vi "RT Loop - Image Acquisition and Processing.vi"(8 "error in (no error)":errorcluster, 9 "FPGA VI Reference":T1, 10 "Vision Cmd Queue":refnum<queue>, 11 "Message Handling Queue":refnum<queue>) -> ()   [LabVIEW 2018]
doc: "Executes the sequence sent from the main UI."
uses:
  controls/Sequence Engine State.ctl
  controls/FPGA VI Reference.ctl
  <vilib>/rvi/interface/nirviReadWriteControl/nirviReadWriteControl.xnode
  NiFpgaLv.dll
  <vilib>/Utility/error.llb/Error Cluster From Error Code.vi
  <vilib>/rvi/interface/Simulation/niFpgaSimulationCallBeginRW.vi
  <vilib>/rvi/errors/niLvFpgaAdjustHostInterfaceError.vi
  support/Message Queue/Message Cluster.ctl
  support/Message Queue/Message Queue.lvlib
  Globals/Global - All RT Loop Stop.vi
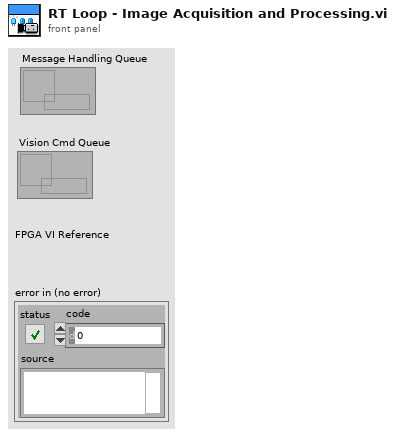
[diagram p1: front panel]
types:
  T1 = typedef "FPGA VI Reference.ctl" = refnum<k20>
  T2 = typedef "Message Queue.lvlib/Message Cluster.ctl" = cluster{"Message":string, "Message Data":variant}
  T3 = typedef "Sequence Engine State.ctl" = enum16{"Idle", "Running", "Stop", "Pause", "Resume", "Load Sequence"}
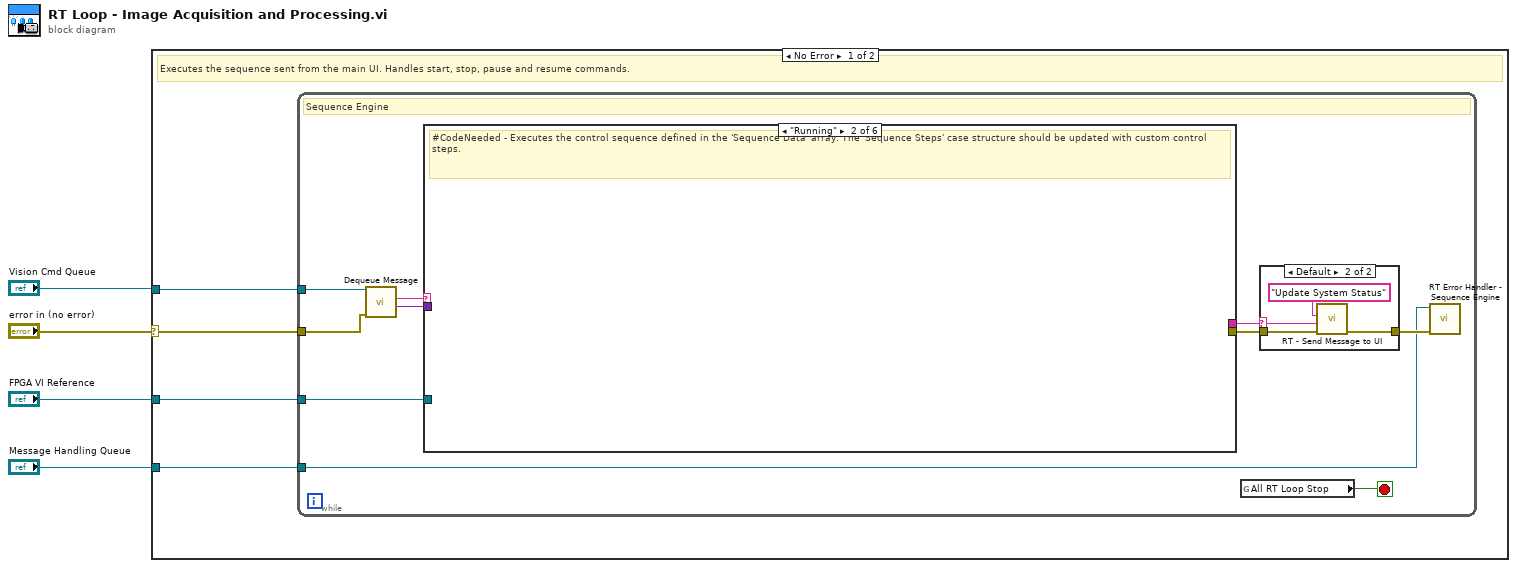
[diagram p0: block diagram]
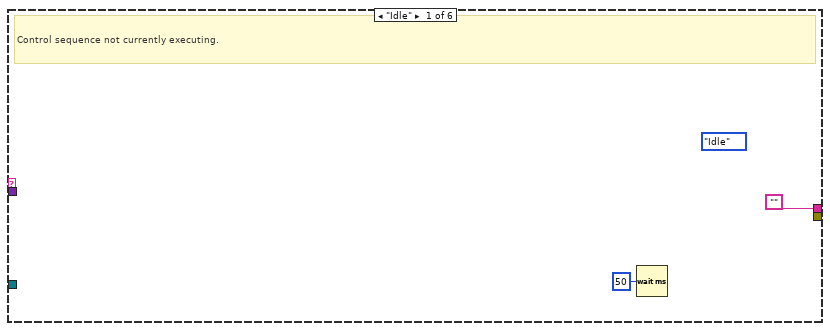
[diagram p3: hidden frame]
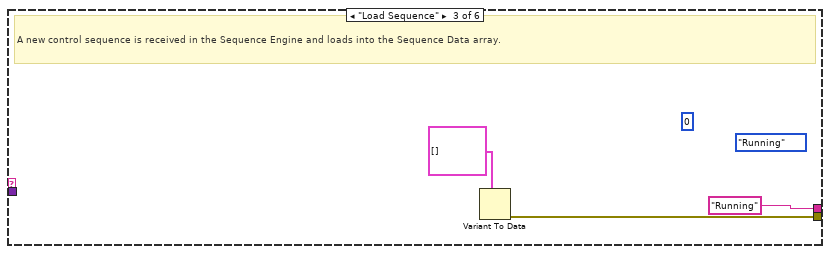
[diagram p4: hidden frame]
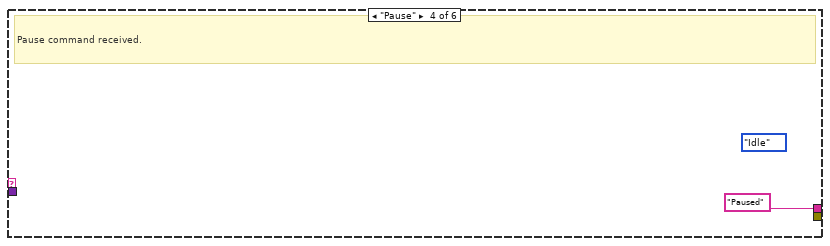
[diagram p5: hidden frame]
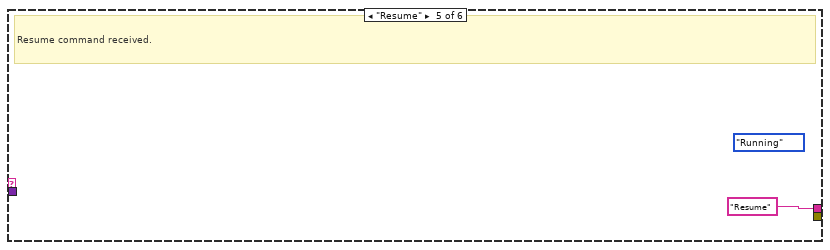
[diagram p6: hidden frame]
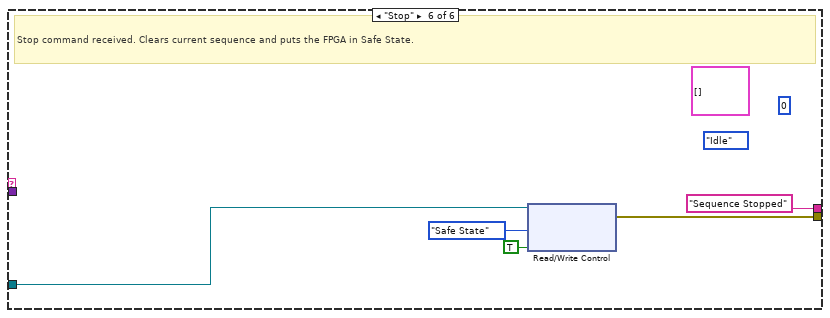
[diagram p7: hidden frame]
diagram:
  n1 = case shown="No Error" "error in (no error)" {
    selector: "error in (no error)" -> [w5 _]
    tunnel: "Message Handling Queue" -> [w8 _]
    tunnel: "Vision Cmd Queue" -> [w7 _]
    tunnel: "FPGA VI Reference" -> [w6 _]
    frame No Error {
      # "Executes the sequence sent from the main UI. Handles start, stop, pause and resume commands."
      n2 = while "Sequence Engine" {
        tunnel: w7 -> [w12]
        tunnel: w6 -> [w18]
        tunnel: w8 -> [w15]
        tunnel: w5 -> [w11]
        stop <- w14 stop-if-true
        # "Sequence Engine"
        n3 = call "Dequeue Message.vi"("error in (no error)"=w11, "Message Queue"=w12) -> ("Message Data"=w9:variant, "Message"=w10:string)  [unwired: 6 in, 2 out]
        n4 = case shown="\"Running\"" w10 {
          tunnel: w18 -> [_ _ _ _ _ w43]
          tunnel: [_ _ w29 _ _ w42] -> w17
          tunnel: ["" ("f") _ "Running" ("f") "Paused" "Resume" ("f") "Sequence Stopped"] -> w13
          tunnel: w9 -> [_ _ _ _ _ _]
          frame "Idle" {
            w25 = Sequence_Engine_State."Idle" ("Sequence Engine State")
            # "Control sequence not currently executing."
            n5 = Wait (ms)(milliseconds to wait=u32 50) -> ()  [unwired: 1 out]
          }
          frame "Running" {
            # "#CodeNeeded - Executes the control sequence defined in the 'Sequence Data' array. The 'Sequence Steps' case structure should be updated with custom control steps."
          }
          frame "Load Sequence" {
            w31 = 0 ("Current Step")
            w30 = Sequence_Engine_State."Running" ("Sequence Engine State")
            # "A new control sequence is received in the Sequence Engine and loads into the Sequence Data array."
            n6 = Variant To Data(type=T2[] []) -> (data=w32:T2[], error out=w29:errorcluster)  [unwired: 2 in]
          }
          frame "Pause" {
            w34 = Sequence_Engine_State."Idle" ("Sequence Engine State")
            # "Pause command received."
          }
          frame "Resume" {
            w36 = Sequence_Engine_State."Running" ("Sequence Engine State")
            # "Resume command received."
          }
          frame "Stop" {
            w38 = 0
            w39 = T2[] []
            w41 = Sequence_Engine_State."Idle" ("Sequence Engine State")
            # "Stop command received. Clears current sequence and puts the FPGA in Safe State."
            n7 = xnode "Read/Write Control"("FPGA VI Reference In"=w43, "New State"=enum16{"Safe State", "Control (PID)"}."Safe State", "Change State"=TRUE) -> ("error out"=w42:errorcluster)  [unwired: 1 in, 1 out]
          }
        }
        n8 = global read "Global - All RT Loop Stop.vi" "All RT Loop Stop"() -> (w14:bool)
        n9 = case shown="Default" w13 {
          selector: w13 -> [_ w20]
          tunnel: w17 -> [w19 w23]
          tunnel: [w19 w21] -> w16
          frame "" {
            # "Blank. Send nothing."
          }
          frame Default {
            n10 = call "RT - Send Message to UI.vi"("error in (no error)"=w23, "Message Data"=w20, "Message"="Update System Status") -> ("error out"=w21:errorcluster)  [unwired: 8 in]
          }
        }
        n11 = call "RT Error Handler - Sequence Engine.vi"("error in (no error)"=w16, "Message Queue"=w15) -> ()  [unwired: 9 in, 1 out]
      }
    }
    frame Error {
      # "Input Error. Do nothing."
    }
  }
